vi "FLIR camera.vi"() -> ()   [LabVIEW 2020]
doc: "The Stream to AVI Files example shows how to save images to an AVI file when using a grab acquisition. This example uses a grab acquisition which works for all camera formats and image sizes. It is recommended to use the Stream to AVI File (Optimized Performance) example if your camera settings work with a ring acquisition."
uses:
  <vilib>/vision/Avi.llb/IMAQ AVI2 Codec Path.ctl
  Program Files (x86)/National Instruments/LabVIEW 2020/examples/Vision Acquisition/NI-IMAQdx/SubVIs/Grab Manager Mode.ctl
  <vilib>/vision/Image Controls.llb/IMAQ Image.ctl
  <vilib>/vision/driver/IMAQdx.llb/IMAQdx Buffer Number Mode.ctl
  <vilib>/Utility/High Resolution Relative Seconds.vi
  <vilib>/vision/driver/NI_Vision_Acquisition_Software.lvlib
  <resource>/objmgr/imaqdx.rc
panel:
  out "Boolean":bool
  out "Image":T1(plugin-control)
  out "stripped path":path
  in  "Skip Count":u32
  out "Images Saved Per Second":dbl
  out "Images Acquired Per Second":dbl
  in  "Images per AVI":i32=100
  out "Write Speed":dbl(graph) caption="Image File Write Speed"
  in  "Start":bool
  in  "Codec":u16(ring) items=["FF Video Codec 1 (FFV1) (NI Vision)", "Motion JPEG (NI Vision)", "VP8 (NI Vision)", "VP9 (NI Vision)", "Y800 Uncompressed Grey Scale (NI Vision)", "YUV 4:2:0 Planar (NI Vision)"]
  out "Destination Folder":path
  out "Images Behind":i32
  in  "Number of Images":u32=30
  in  "Camera Name":refnum<k21> caption="IMAQdx Session"
  in  "Stop":bool
  # "Overview: Demonstrates how to stream images to an AVI file when using a grab acquisition.\nRequirements: Vision Acquisition Software\nInstructions:\n1. Select the Camera Name\n2. Run the VI\n3. Select the Codec and click Start.\n4. Increase the Skip Count if Images Behind is greater than 0."
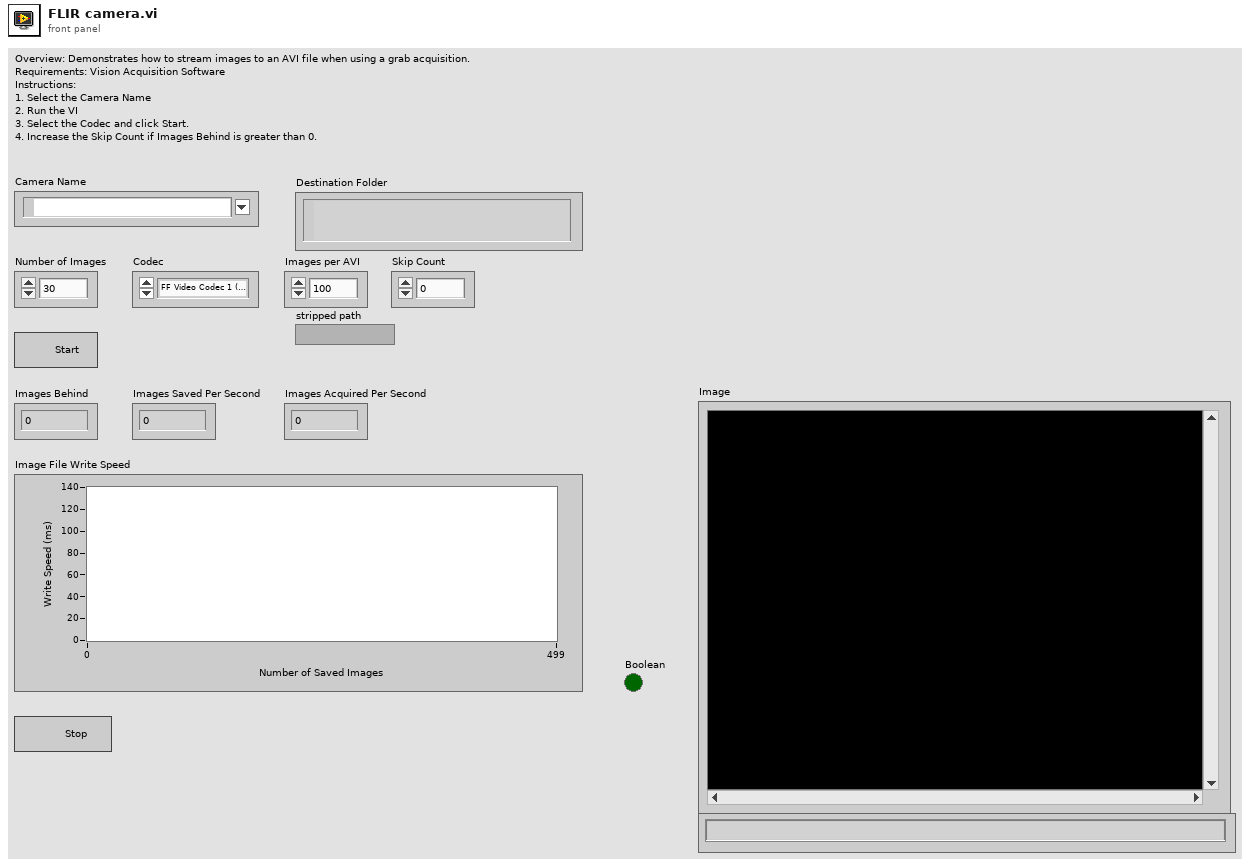
[diagram p1: front panel]
types:
  T1 = typedef "IMAQ Image.ctl" = refnum<image>
  T2 = typedef "IMAQ AVI2 Codec Path.ctl" = u32
  T3 = typedef "IMAQdx.ctl" = refnum<k21>
  T4 = typedef "Grab Manager Mode.ctl" = enum16{"Create Processing Images", "Lock", "Add Acquired Image", "Get Acquired Image", "Unlock", "Dispose Processing Images"}
  T5 = cluster{"Number of Processing Images":u32, "Image Border Size":u32}
  T6 = typedef "NI_Vision_Acquisition_Software.lvlib/IMAQdx Buffer Number Mode.ctl" = enum32{"Next", "Last", "Buffer Number", "Every", "Last New"}
  T7 = typedef "IMAQ AVI2 Refnum.ctl" = refnum<k20>
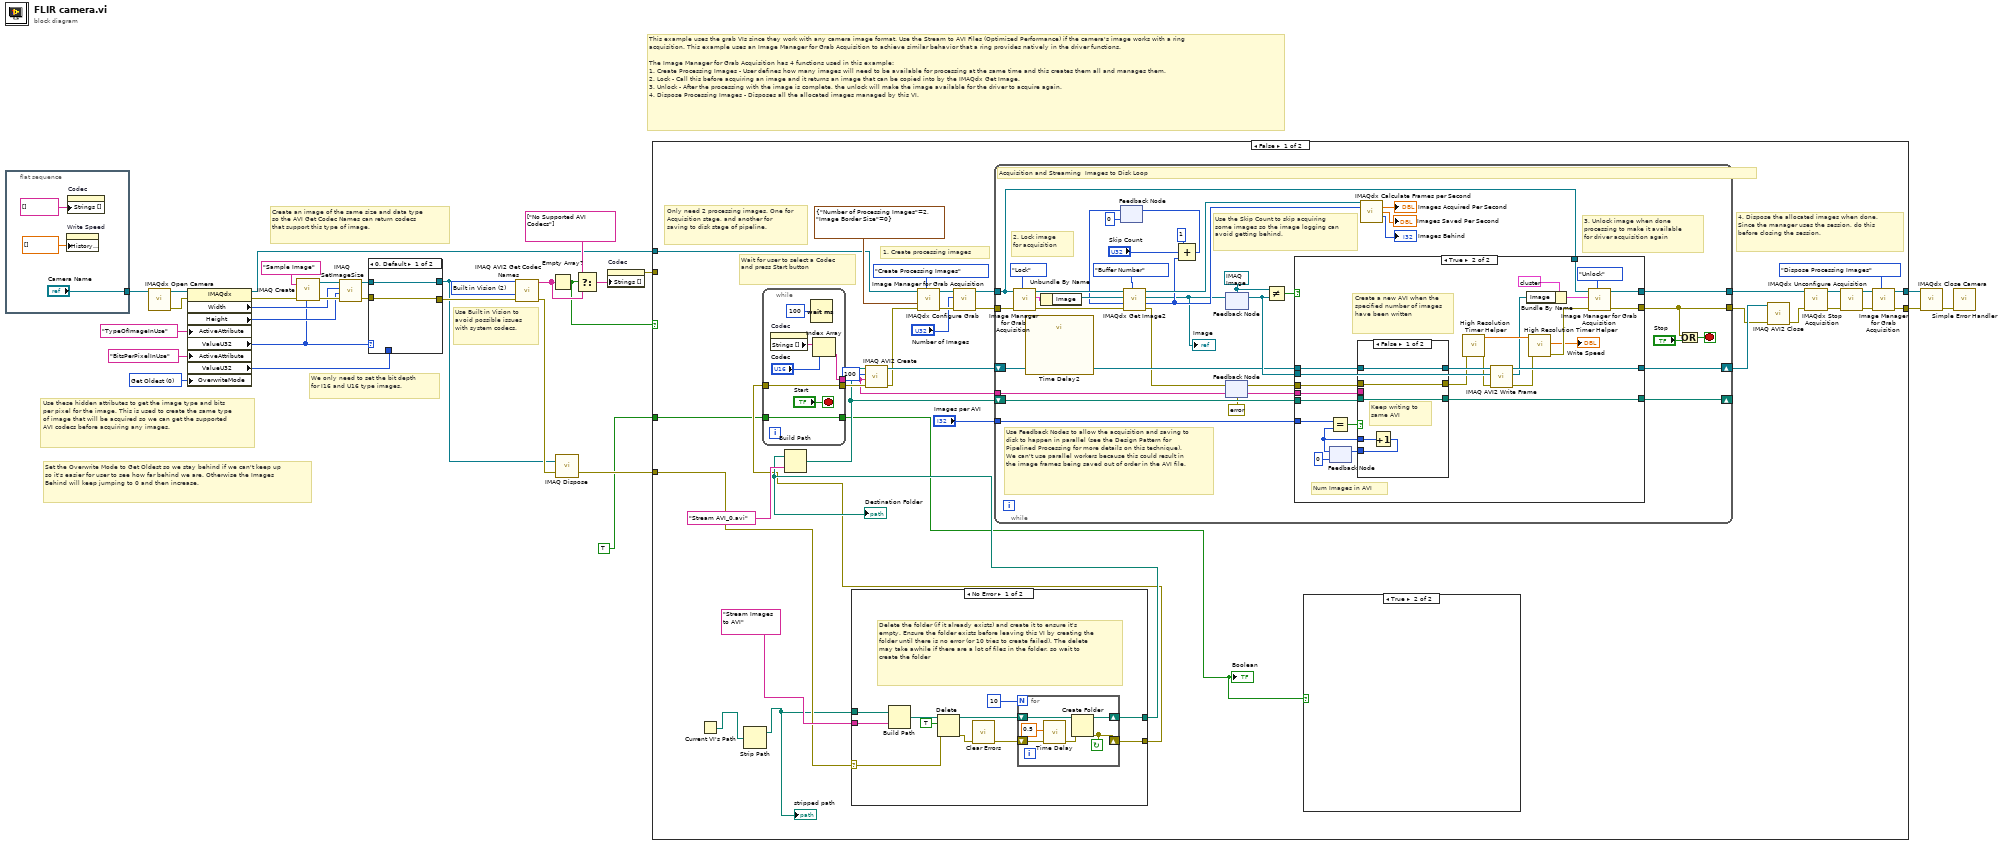
[diagram p0: block diagram]
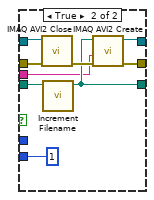
[diagram p5: hidden frame]
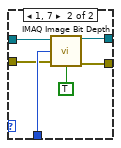
[diagram p7: hidden frame]
diagram:
  w2 = T2 2 items=["Default", "System", "Built in Vision"] ("Codec Source")
  w4 = u32 0 items=["Get Oldest"=0, "Fail"=2, "Get Newest"=3] ("OverwriteMode")
  # "Use Built in Vision to avoid possible issues with system codecs."
  # "This example uses the grab VIs since they work with any camera image format. Use the Stream to AVI Files (Optimized Performance) if the camera's image works with a ring acquisition. This example uses an Image Manager for Grab Acquisition to achieve similar behavior that a ring provides natively in the driver functions.\n\nThe Image Manager for Grab Acquisition has 4 functions used in this example:\n1. Create Processing Images - User defines how many images will need to be available for processing at the same time and this creates them all and manages them.\n2. Lock - Call this before acquiring an image and it returns an image that can be copied into by the IMAQdx Get Image.\n3. Unlock - After the processing with the image is complete, the unlock will make the image available for the driver to acquire again.\n4. Dispose Processing Images - Disposes all the allocated images managed by this VI."
  # "Set the Overwrite Mode to Get Oldest so we stay behind if we can't keep up so it's easier for user to see how far behind we are. Otherwise the Images Behind will keep jumping to 0 and then increase."
  # "Create an image of the same size and data type so the AVI Get Codec Names can return codecs that support this type of image."
  # "Use these hidden attributes to get the image type and bits per pixel for the image. This is used to create the same type of image that will be acquired so we can get the supported AVI codecs before acquiring any images."
  # "We only need to set the bit depth for I16 and U16 type images."
  n1 = flat-sequence {
    tunnel: ["Camera Name"] -> w31
    frame #0 {
      n2 = property on="Write Speed" class="WFChart (strict)"("History Data"=dbl[] []) -> ()  [unwired: 2 in, 2 out]
      n3 = property on="Codec" class="Ring (strict)"("Strings []"=string[] []) -> ()  [unwired: 2 in, 2 out]
    }
  }
  n4 = call <vilib>:"IMAQdx Open Camera.vi"("Session In"=w31) -> ("error out"=w27:errorcluster, "Session Out"=w28:T3)  [unwired: 2 in, 7 out]
  n5 = property class="IMAQdx"(reference=w28, error in=w27, "ActiveAttribute"="TypeOfImageInUse", "ActiveAttribute"="BitsPerPixelInUse", "OverwriteMode"=w4) -> (reference out=w13:T3, error out=w25:errorcluster, "Width"=w21:u32, "Height"=w20:u32, "ValueU32"=w8:u32, "ValueU32"=w11:u32)
  n6 = call "IMAQ Create"("Image Name"="Sample Image", "Image Type"=w8, "error in (no error)"=w25) -> ("New Image"=w22:T1, "error out"=w23:errorcluster)  [unwired: 1 in, 1 out]
  n7 = call "IMAQ SetImageSize"("error in (no error)"=w23, "Y Resolution"=w20, "X Resolution"=w21, "Image"=w22) -> ("error out"=w10:errorcluster, "Image Out"=w9:T1)  [unwired: 1 in]
  n8 = case shown="0, Default" w8 {
    tunnel: [w35 w42] -> w14
    tunnel: w11 -> [_ w41]
    tunnel: w10 -> [w35 w40]
    tunnel: w9 -> [w36 w38]
    tunnel: [w36 w37] -> w5
    frame 0, Default {
    }
    frame 1, 7 {
      n9 = call "IMAQ Image Bit Depth"("Image"=w38, "Bit Depth (0)"=w41, "error in (no error)"=w40, "Get/Set Bit Depth? (Set)"=TRUE) -> ("Image Out"=w37:T1, "error out"=w42:errorcluster)  [unwired: 9 in, 1 out]
    }
  }
  n10 = call "IMAQ AVI2 Get Codec Names"("error in (no error)"=w14, "Codec Source"=w2, "Image"=w5) -> ("error out"=w7:errorcluster, "Codec Names"=w19:string[])  [unwired: 7 in]
  n11 = Empty Array?(array=w19) -> (empty?=w15:bool)
  n12 = call "IMAQ Dispose"("Image"=w5, "error in (no error)"=w7) -> ("error out"=w6:errorcluster)  [unwired: 4 in]
  n13 = Select(t=string[] ["No Supported AVI Codecs"], s=w15, f=w19) -> (s? t:f=w17:string[])
  n14 = property on="Codec" class="Ring (strict)"("Strings []"=w17) -> (error out=w16:errorcluster)  [unwired: 2 in, 1 out]
  n15 = case shown="False" w15 {
    tunnel: [w53 w182] -> w30
    tunnel: [w54 w183] -> w29
    tunnel: w13 -> [w59 w183]
    tunnel: w6 -> [w50 w182]
    tunnel: w16 -> [_ _]
    tunnel: TRUE -> [w45 _]
    frame False {
      # "4. Dispose the allocated images when done. Since the manager uses the session, do this before closing the session."
      # "1. Create processing images"
      # "Only need 2 processing images. One for Acquisition stage, and another for saving to disk stage of pipeline."
      # "Wait for user to select a Codec and press Start button"
      n16 = Current VI's Path() -> (path=w47:path)
      n17 = Strip Path(path=w47) -> (stripped path=w46:path)  [unwired: 1 out]
      "stripped path" <- w46
      n18 = case shown="No Error" w50 {
        selector: w50 -> [w79 w95]
        tunnel: w46 -> [w88 _]
        tunnel: [w81 _] -> w49
        tunnel: "Stream Images to AVI" ("Folder Name") -> [w80 _]
        tunnel: [w78 w95] -> w48
        frame No Error {
          # "Delete the folder (if it already exists) and create it to ensure it's empty. Ensure the folder exists before leaving this VI by creating the folder until there is no error (or 10 tries to create failed). The delete may take awhile if there are a lot of files in the folder, so wait to create the folder"
          n19 = Build Path(base path=w88, name or relative path=w80) -> (appended path=w86:path)
          n20 = Delete(path (use dialog)=w86, entire hierarchy (F)=TRUE, error in=w79) -> (deleted path=w85:path, error out=w84:errorcluster)  [unwired: 2 in, 1 out]
          n21 = call <vilib>:"Clear Errors.vi"("error in (no error)"=w84) -> ("error out"=w83:errorcluster)  [unwired: 5 in, 1 out]
          n22 = for {
            N: 10 -> [_]
            shift-right: [w93] -> w81
            shift-left: w85 -> [w94]
            shift-right: [w92] -> w78
            shift-left: w83 -> [w91]
            stop <- w92 continue-if-true
            n23 = call "Time Delay"("error in (no error)"=w91, "Delay Time (s)"=0.5) -> ("error out"=w90:errorcluster)  [unwired: 9 in]
            n24 = Create Folder(path (use dialog)=w94, error in=w90) -> (created path=w93:path, error out=w92:errorcluster)  [unwired: 2 out]
          }
        }
        frame Error {
        }
      }
      "Destination Folder" <- w49
      n25 = while {
        tunnel: w48 -> [w180]
        tunnel: [w180] -> w74
        tunnel: [w177] -> w66
        tunnel: [w175] -> w44
        tunnel: w45 -> [w175]
        stop <- "Start" stop-if-true
        n26 = property on="Codec" class="Ring (strict)"() -> ("Strings []"=w178:string[])  [unwired: 2 in, 2 out]
        n27 = Wait (ms)(milliseconds to wait=u32 100) -> ()  [unwired: 1 out]
        n28 = Index Array(array=w178, index="Codec") -> (element=w177:string)
      }
      "Boolean" <- w44
      n29 = Build Path(base path=w49, name or relative path="Stream AVI_0.avi") -> (appended path=w67:path)
      n30 = call "IMAQ AVI2 Create"("error in (no error)"=w74, "Codec"=w66, "Frames Per Second"=u32 100, "AVI Path"=w67) -> ("error out"=w58:errorcluster, "AVI Refnum"=w69:T7)  [unwired: 6 in]
      n31 = call "Image Manager for Grab Acquisition.vi"("Mode"=Grab_Manager_Mode."Create Processing Images", "error in (no error)"=w58, "Init Settings"=T5 {"Number of Processing Images"=2, "Image Border Size"=0}, "Session In"=w59) -> ("error out"=w61:errorcluster, "Session Out"=w60:T3)  [unwired: 4 in, 2 out]
      n32 = call <vilib>:"IMAQdx Configure Grab.vi"("error in"=w61, "Number of Buffers"="Number of Images", "Session In"=w60) -> ("error out"=w64:errorcluster, "Session Out"=w65:T3)  [unwired: 7 in]
      n33 = while {
        tunnel: w64 -> [w113]
        tunnel: w65 -> [w114]
        tunnel: [w128] -> w75
        tunnel: [w121] -> w72
        shift-right: [w129] -> w73
        shift-left: w69 -> [w120]
        tunnel: "Images per AVI" -> [w116]
        shift-right: [w117] -> _
        shift-left: w67 -> [w118]
        tunnel: w66 -> [w119]
        stop <- w123 stop-if-true
        w126 = T1 refnum ("Image Out")
        # "3. Unlock image when done processing to make it available for driver acquisition again"
        # "2. Lock image for acquisition"
        # "Use the Skip Count to skip acquiring some images so the image logging can avoid getting behind."
        # "Use Feedback Nodes to allow the acquisition and saving to disk to happen in parallel (see the Design Pattern for Pipelined Processing for more details on this technique). We can't use parallel workers because this could result in the image frames being saved out of order in the AVI file."
        # "Acquisition and Streaming  Images to Disk Loop"
        n34 = call "Image Manager for Grab Acquisition.vi"("Mode"=Grab_Manager_Mode."Lock", "error in (no error)"=w113, "Session In"=w114) -> ("error out"=w110:errorcluster, "Image Settings Out"=w108:cluster{"Image":T1, "Buffer Number":u32}, "Session Out"=w111:T3)  [unwired: 5 in, 1 out]
        n35 = call "Time Delay2"() -> ()  [unwired: 11 in, 1 out]
        n36 = Unbundle By Name(w108) -> ("Image"=w107:T1)
        n37 = feedback #1(u32 0) -> (w104:u32)
        n38 = call <vilib>:"IMAQdx Get Image2.vi"("Buffer Number Mode (Next)"=IMAQdx_Buffer_Number_Mode."Buffer Number", "error in"=w110, "Buffer Number In"=w104, "Image In"=w107, "Session In"=w111) -> ("error out"=w106:errorcluster, "Buffer Number Out"=w100:u32, "Image Out"=w96:T1, "Session Out"=w105:T3)  [unwired: 3 in]
        "Image" <- w96
        n39 = Compound Arithmetic op=ADD(u32 1, "Skip Count", w100) -> (w99:u32)
        n40 = feedback-in #1(w99) -> ()
        n41 = feedback-in #2(w106) -> ()
        n42 = feedback #2(errorcluster {"status"=FALSE, "code"=0, "source"=""} ("error out")) -> (w127:errorcluster)
        n43 = feedback-in #3(w96) -> ()
        n44 = feedback #3(w126) -> (w124:T1)
        n45 = Not Equal?(x=w126, y=w124) -> (x != y?=w125:bool)
        n46 = case shown="True" w125 {
          tunnel: w120 -> [w132 w155]
          tunnel: w124 -> [_ w149]
          tunnel: w127 -> [w133 w154]
          tunnel: [w132 w160] -> w129
          tunnel: [w134 w143] -> w128
          tunnel: w114 -> [w134 w140]
          tunnel: [w133 w142] -> w121
          tunnel: w119 -> [_ w153]
          tunnel: w118 -> [w131 w152]
          tunnel: [w131 w150] -> w117
          tunnel: w116 -> [_ w148]
          frame False {
            # "First iteration doesn't have valid image for this pipelined stage."
          }
          frame True {
            # "Create a new AVI when the specified number of images have been written"
            # "Num Images in AVI"
            n47 = feedback #4(0) -> (w159:i32)
            n48 = Equal?(x=w148, y=w159) -> (x = y?=w156:bool)
            n49 = case shown="False" w156 {
              tunnel: [w164 1] -> w158
              tunnel: w159 -> [w165 _]
              tunnel: w155 -> [w163 w172]
              tunnel: [w163 w169] -> w151
              tunnel: w152 -> [w161 w173]
              tunnel: w154 -> [w162 w171]
              tunnel: [w162 w168] -> w147
              tunnel: [w161 w167] -> w150
              tunnel: w153 -> [_ w166]
              frame False {
                # "Keep writing to same AVI"
                n50 = Increment(x=w165) -> (x+1=w164:i32)
              }
              frame True {
                n51 = call "IMAQ AVI2 Close"("error in (no error)"=w171, "AVI Refnum"=w172) -> ("error out"=w170:errorcluster)  [unwired: 9 in]
                n52 = call "Increment Filename.vi"("Path In"=w173) -> ("Incremented Path Out"=w167:path)  [unwired: 10 in]
                n53 = call "IMAQ AVI2 Create"("error in (no error)"=w170, "Codec"=w166, "AVI Path"=w167) -> ("error out"=w168:errorcluster, "AVI Refnum"=w169:T7)  [unwired: 7 in]
              }
            }
            n54 = feedback-in #4(w158) -> ()
            n55 = call "High Resolution Timer Helper.vi"("error in (no error)"=w147) -> ("error out"=w146:errorcluster, "Current Time"=w144:dbl)  [unwired: 8 in, 1 out]
            n56 = call "IMAQ AVI2 Write Frame"("error in (no error)"=w146, "Image"=w149, "AVI Refnum"=w151) -> ("error out"=w145:errorcluster, "Image Out (duplicate)"=w137:T1, "AVI Refnum (duplicate)"=w160:T7)  [unwired: 6 in]
            n57 = Bundle By Name(cluster=cluster{"Image":T1, "Buffer Number":u32} {"Image"=refnum, "Buffer Number"=0} ("Image Settings In"), "Image"=w137) -> (w136:cluster{"Image":T1, "Buffer Number":u32})
            n58 = call "High Resolution Timer Helper.vi"("error in (no error)"=w145, "Previous Time"=w144) -> ("error out"=w141:errorcluster, "Time Difference (ms)"=→"Write Speed":dbl)  [unwired: 7 in, 1 out]
            n59 = call "Image Manager for Grab Acquisition.vi"("Mode"=Grab_Manager_Mode."Unlock", "error in (no error)"=w141, "Image Settings In"=w136, "Session In"=w140) -> ("error out"=w142:errorcluster, "Session Out"=w143:T3)  [unwired: 4 in, 2 out]
          }
        }
        n60 = call <vilib>:"IMAQdx Calculate Frames per Second.vi"("Session In"=w105, "Buffer Number"=w100) -> ("Acquired Frames per Second"=→"Images Acquired Per Second":dbl, "Processed Frames per Second"=→"Images Saved Per Second":dbl, "Images Behind"=→"Images Behind":i32)  [unwired: 7 in, 4 out]
        n61 = Or(x=w121, y="Stop") -> (x .or. y?=w123:bool)
      }
      n62 = case shown="True" w44 {
        frame False {
        }
        frame True {
        }
      }
      n63 = call "IMAQ AVI2 Close"("error in (no error)"=w72, "AVI Refnum"=w73) -> ("error out"=w71:errorcluster)  [unwired: 9 in]
      n64 = call <vilib>:"IMAQdx Stop Acquisition.vi"("error in"=w71, "Session In"=w75) -> ("error out"=w76:errorcluster, "Session Out"=w77:T3)  [unwired: 8 out]
      n65 = call <vilib>:"IMAQdx Unconfigure Acquisition.vi"("error in"=w76, "Session In"=w77) -> ("error out"=w57:errorcluster, "Session Out"=w56:T3)  [unwired: 8 out]
      n66 = call "Image Manager for Grab Acquisition.vi"("Mode"=Grab_Manager_Mode."Dispose Processing Images", "error in (no error)"=w57, "Session In"=w56) -> ("error out"=w53:errorcluster, "Session Out"=w54:T3)  [unwired: 5 in, 2 out]
    }
    frame True {
      # "No valid AVI Codecs for the image size and image type."
    }
  }
  n67 = call <vilib>:"IMAQdx Close Camera.vi"("error in"=w30, "Session In"=w29) -> ("error out"=w3:errorcluster)  [unwired: 9 out]
  n68 = call <vilib>:"Simple Error Handler.vi"("error in (no error)"=w3) -> ()  [unwired: 4 in, 5 out]
